vi "OpenLabVIEW.vi"(1 "Port":u16=3364, 2 "Address":string="localhost") -> (0 "LabVIEW":refnum<vi>)   [LabVIEW 2014]
uses:
  LabVIEW.vi
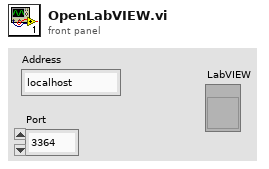
[diagram p1: front panel]
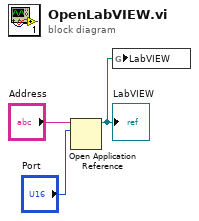
[diagram p0: block diagram]
diagram:
  n1 = Open Application Reference(10:"Port", 11:"Address") -> (3:w1:refnum<vi>)  [unwired: 2 in, 1 out]
  "LabVIEW" <- w1
  n2 = global write "LabVIEW.vi" "LabVIEW"(w1) -> ()
